vi "Match.vi"(0 "Number to Match":i32=50 min=0 max=1000) -> (1 "Number of Interactions":i32, 2 "Current Number":dbl)   [LabVIEW 2016]
doc: "Este VI consiste en encontrar un cierto numero dado de manera aleatoria en un rango de 0-1000 con la ayuda de un while-loop"
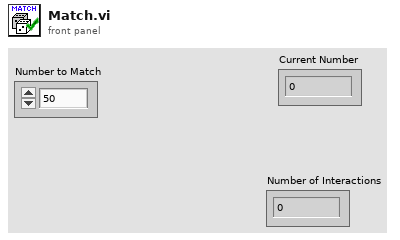
[diagram p1: front panel]
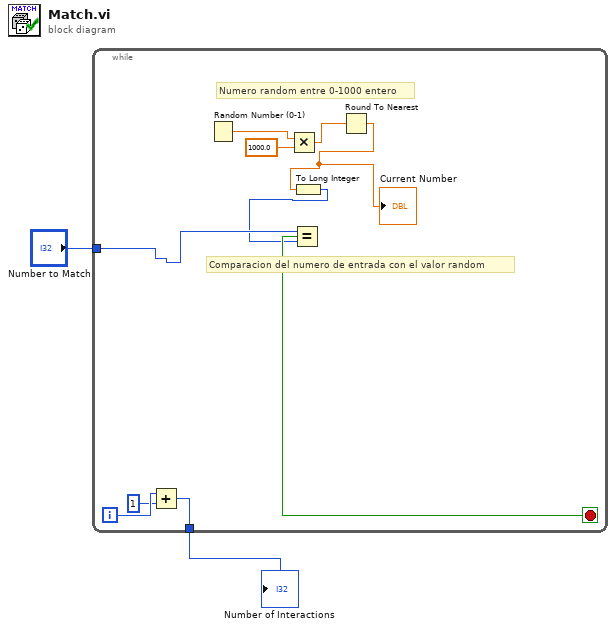
[diagram p0: block diagram]
diagram:
  n1 = while {
    tunnel: "Number to Match" -> [w8]
    tunnel: [w5] -> w1
    i -> [w7]
    stop <- w9 stop-if-true
    # "Comparacion del numero de entrada con el valor random"
    # "Numero random entre 0-1000 entero"
    n2 = Add(x=w7, y=1) -> (x+y=w5:i32)
    n3 = Random Number (0-1)() -> (number: 0 to 1=w12:dbl)
    n4 = Multiply(x=w12, y=1000.0) -> (x*y=w10:dbl)
    n5 = Round To Nearest(number=w10) -> (nearest integer value=w4:dbl)
    "Current Number" <- w4
    n6 = To Long Integer(number=w4) -> (32bit integer=w3:i32)
    n7 = Equal?(x=w8, y=w3) -> (x = y?=w9:bool)
  }
  "Number of Interactions" <- w1
